vi "toplinegrabber.vi"(7 "error in":errorcluster) -> (27 "error out":errorcluster)   [LabVIEW 2011]
uses:
  <vilib>/vision/NI_Vision_Development_Module.lvlib
panel:
  out "Image Out":T1(plugin-control)
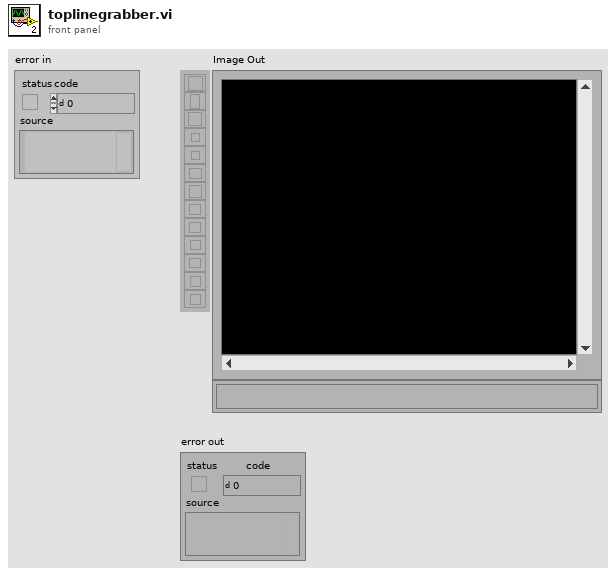
[diagram p1: front panel]
types:
  T1 = typedef "IMAQ Image.ctl" = refnum<image>
  T2 = cluster{"Show Search Area":bool, "Show Search Lines":bool, "Show Edges Found":bool, "Show Result":bool}
  T3 = cluster{"Number of Lines":i32, "Type":enum32{"First Edge Rake", "Best Edge Rake", "Hough Edge Rake", "First Edge Projection", "Best Edge Projection"}, "Min. Score":dbl, "Max. Score":dbl, "Orientation":dbl, "Angle Range":dbl, "Angle Tolerance":dbl, "Step Size":u32, "Min. SNR (db)":dbl, "Min. Points (%)":dbl, "Hough Iterations":i32}
  T4 = cluster{"Edge Polarity":u32, "Kernel Size":u32, "Width":u32, "Minimum Edge Strength":sgl, "Interpolation Type":enum32{"Zero Order", "Bilinear", "Quadratic", "Cubic", "Bilinear Fixed"}, "Data Processing Method":enum32{"Average", "Median"}}
  T5 = cluster{"Global Rectangle":i32[], "Contours":cluster{"ID":enum32{"External", "Internal"}, "Type":u32, "Coordinates":i32[]}[]}
  T6 = typedef "Image Type" = u32
  T7 = cluster{"Point1 (Pixels)":cluster{"X":sgl, "Y":sgl}, "Point2 (Pixels)":cluster{"X":sgl, "Y":sgl}, "Point1 (Real-World)":cluster{"X":sgl, "Y":sgl}, "Point2 (Real-World)":cluster{"X":sgl, "Y":sgl}, "Angle (Pixel)":dbl, "Angle (Real-World)":dbl, "Score":dbl, "Straightness":dbl, "Average SNR (db)":dbl, "Calibration Valid":bool}[]
  T8 = typedef "Search Line.ctl" = cluster{"Start Point":cluster{"X":sgl, "Y":sgl}, "End Point":cluster{"X":sgl, "Y":sgl}, "Edge Info":T9[], "Edge Map":dbl[], "Calibration Valid":bool}
  T9 = typedef "Edge New.ctl" = cluster{"Location (Pixel)":cluster{"X":sgl, "Y":sgl}, "Location (Real-World)":cluster{"X":sgl, "Y":sgl}, "Distance (Pixel)":dbl, "Distance (Real-World)":dbl, "Strength":dbl, "Noise":dbl, "Rising?":bool}
  T10 = cluster{"Straight Edges":cluster{"Point1 (Pixels)":cluster{"X":sgl, "Y":sgl}, "Point2 (Pixels)":cluster{"X":sgl, "Y":sgl}, "Point1 (Real-World)":cluster{"X":sgl, "Y":sgl}, "Point2 (Real-World)":cluster{"X":sgl, "Y":sgl}, "Angle (Pixel)":dbl, "Angle (Real-World)":dbl, "Score":dbl, "Straightness":dbl, "Average SNR (db)":dbl, "Calibration Valid":bool}[], "Search Lines Information":T8[], "Used Edges":cluster{"Edge Information":T9[]}[]}
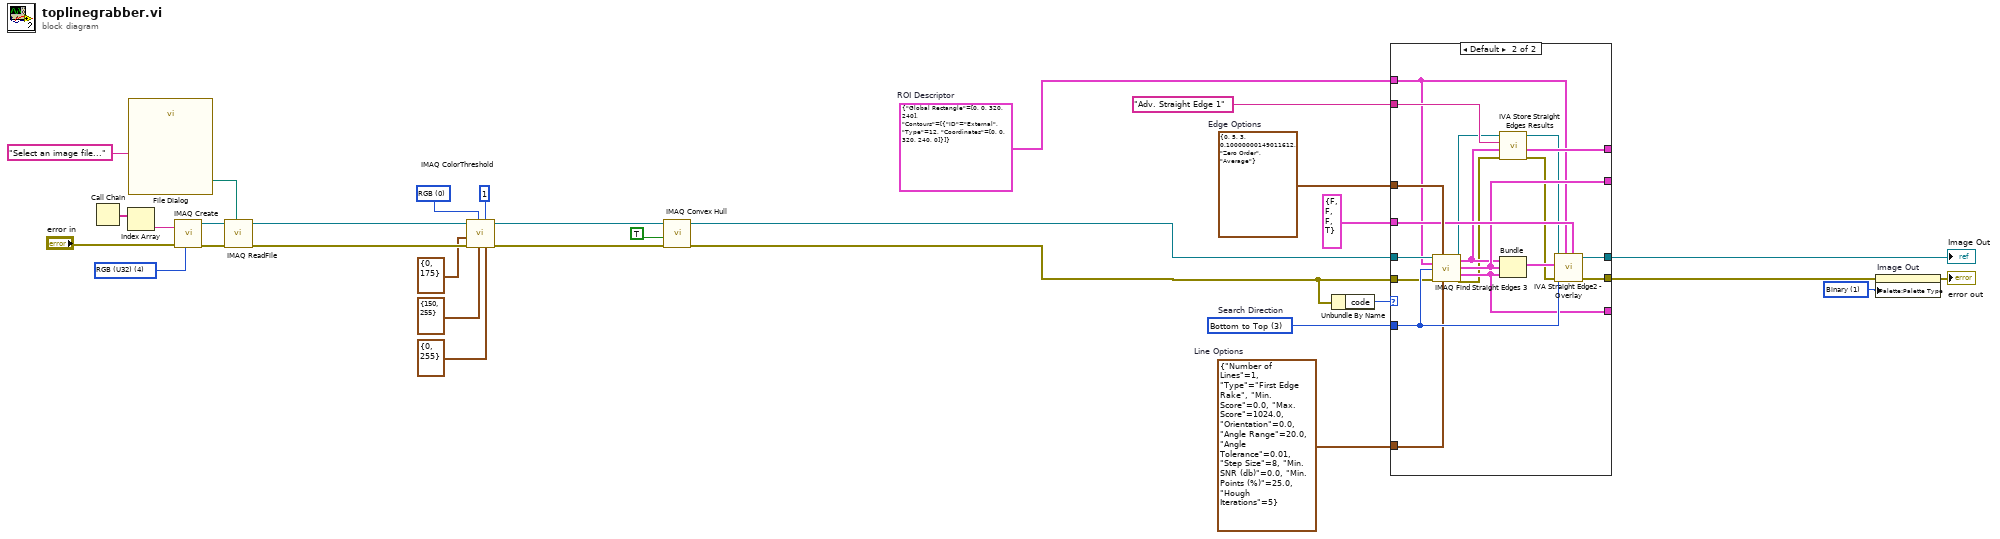
[diagram p0: block diagram]
diagram:
  w2 = u32 1 items=["Grayscale", "Binary", "Gradient", "Rainbow", "Temperature", "User Defined"] ("Palette")
  w10 = T3 {"Number of Lines"=1, "Type"=enum."First Edge Rake", "Min. Score"=0.0, "Max. Score"=1024.0, "Orientation"=0.0, "Angle Range"=20.0, "Angle Tolerance"=0.01, "Step Size"=8, "Min. SNR (db)"=0.0, "Min. Points (%)"=25.0, "Hough Iterations"=5}  # Line Options
  w11 = u32 3 items=["Left to Right", "Right to Left", "Top to Bottom", "Bottom to Top"]  # Search Direction
  w12 = T4 {"Edge Polarity"=0, "Kernel Size"=5, "Width"=3, "Minimum Edge Strength"=0.1, "Interpolation Type"=enum."Zero Order", "Data Processing Method"=enum."Average"}  # Edge Options
  w5 = T5 {"Global Rectangle"=[0, 0, 320, 240], "Contours"=[{"ID"=enum."External", "Type"=12, "Coordinates"=[0, 0, 320, 240, 0]}]}  # ROI Descriptor
  w21 = u16 0 items=["RGB", "HSL", "HSV", "HSI"] ("Color Mode")
  w23 = T6 4 items=["Grayscale (U8)", "Grayscale (I16)", "Grayscale (SGL)", "Complex (CSG)", "RGB (U32)", "HSL (U32)", "RGB (U64)", "Grayscale (U16)"] ("Image Type")
  n1 = Call Chain() -> (call chain=w27:string[])
  n2 = Index Array(array=w27) -> (element=w26:string)  [unwired: 1 in]
  n3 = call "File Dialog"("prompt"="Select an image file...") -> ("selected path"=w24:path)  [unwired: 6 in, 8 out]
  n4 = call "IMAQ Create"("Image Name"=w26, "Image Type"=w23, "error in (no error)"="error in") -> ("New Image"=w30:T1, "error out"=w29:errorcluster)  [unwired: 1 in, 1 out]
  n5 = call "IMAQ ReadFile"("File Path"=w24, "error in (no error)"=w29, "Image"=w30) -> ("error out"=w31:errorcluster, "Image Out"=w17:T1)  [unwired: 2 in, 5 out]
  n6 = call "IMAQ ColorThreshold"("Blue or Luma or Val or Inten Range"=cluster{"Lower value":i32, "Upper value":i32} {"Lower value"=0, "Upper value"=255}, "Replace Value"=1, "Green or Sat Range"=cluster{"Lower value":i32, "Upper value":i32} {"Lower value"=150, "Upper value"=255}, "Color Mode"=w21, "error in (no error)"=w31, "Red or Hue Range"=cluster{"Lower value":i32, "Upper value":i32} {"Lower value"=0, "Upper value"=175}, "Image Src"=w17) -> ("error out"=w16:errorcluster, "Image Dst Out"=w15:T1)  [unwired: 1 in, 2 out]
  n7 = call "IMAQ Convex Hull"("error in (no error)"=w16, "Connectivity 4/8 (8)"=TRUE, "Image Src"=w15) -> ("error out"=w13:errorcluster, "Image Dst Out"=w9:T1)  [unwired: 1 in, 6 out]
  n8 = Unbundle By Name(w13) -> ("code"=w4:i32)
  n9 = case shown="Default" w4 {
    tunnel: w12 -> [_ w51]
    tunnel: w11 -> [_ w50]
    tunnel: w10 -> [_ w49]
    tunnel: w9 -> [w32 w47]
    tunnel: [w32 w46] -> w3
    tunnel: [_ w45] -> w8
    tunnel: T2 {"Show Search Area"=FALSE, "Show Search Lines"=FALSE, "Show Edges Found"=FALSE, "Show Result"=TRUE} ("Setup") -> [_ w44]
    tunnel: w13 -> [_ w43]
    tunnel: [_ w42] -> _
    tunnel: [_ w41] -> _
    tunnel: "Adv. Straight Edge 1" ("Step Name") -> [_ w40]
    tunnel: [_ w39] -> _
    tunnel: w5 -> [_ w37]
    frame -1074396199, -1074396198 {
      # "Discard Coordinate System Error"
    }
    frame Default {
      n10 = call "IMAQ Find Straight Edges 3"("Image"=w47, "Edge Options"=w51, "ROI Descriptor"=w37, "Search Direction"=w50, "error in (no error)"=w43, "Line Options"=w49) -> ("Image (duplicate)"=w36:T1, "Straight Edges"=w38:T7, "Search Lines Information"=w41:T8[], "Used Edges"=w42:cluster{"Edge Information":T9[]}[], "error out"=w34:errorcluster)  [unwired: 1 in, 4 out]
      n11 = call <vilib>:"IVA Store Straight Edges Results.vi"("error in (no error)"=w34, "Straight Edges"=w38, "Step Name"=w40, "Image in"=w36) -> ("error out"=w33:errorcluster, "Straight Edges dup"=w39:T7, "Image dup"=w35:T1)  [unwired: 5 out]
      n12 = Bundle("Straight Edges"=w38, "Search Lines Information"=w41, "Used Edges"=w42) -> (w48:T10)  [unwired: 1 out]
      n13 = call <vilib>:"IVA Straight Edge2 - Overlay.vi"("Setup"=w44, "Search Area"=w37, "error in (no error)"=w33, "Scan Direction"=w50, "Edge Results"=w48, "Image In"=w35) -> ("error out"=w45:errorcluster, "Image Out"=w46:T1)  [unwired: 1 in, 3 out]
    }
  }
  "Image Out" <- w3
  n14 = property on="Image Out" class="ImageControl"(error in=w8, "Palette:Palette Type"=w2) -> (error out=→"error out":errorcluster)  [unwired: 1 in, 1 out]
